vi "FRAS Module CdG.vi"(7 "error in":errorcluster, 8 "Imagette seuillée":i16[][](array[numeric]), 9 "inCdG[Pixels]":dbl[](array[numeric]), 10 "Mode CdG":T1(ring)=enum."Calcul CdG a") -> (0 "error out":errorcluster, 3 "CdGOut [Pixels]":dbl[](array[numeric]))   [LabVIEW 2020]
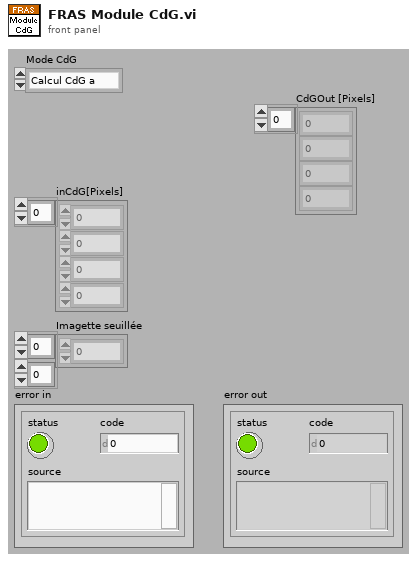
[diagram p1: front panel]
types:
  T1 = enum16{"Initialisation", "Calcul CdG a", "Calcul CdG b"}
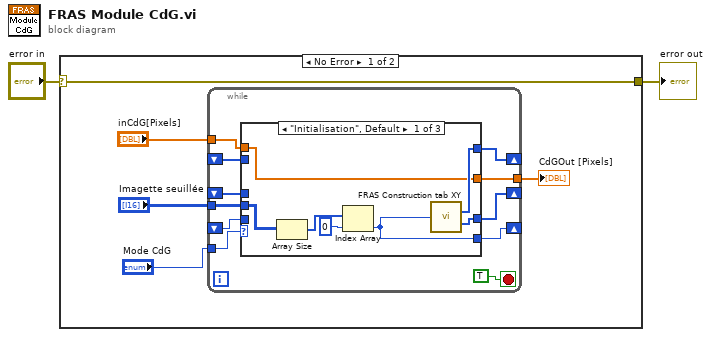
[diagram p0: block diagram]
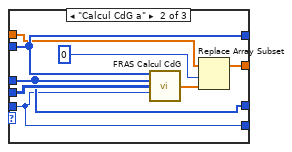
[diagram p2: hidden frame]
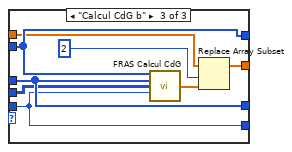
[diagram p3: hidden frame]
diagram:
  n1 = case shown="No Error" "error in" {
    selector: "error in" -> [w3 w42]
    tunnel: [w3 w42] -> w1
    frame No Error {
      n2 = while {
        tunnel: [w18] -> w7
        tunnel: "Imagette seuillée" -> [w17]
        tunnel: "Mode CdG" -> [w15]
        shift-right: [w14] -> _
        shift-left: _ -> [w12]
        shift-right: [w13] -> _
        shift-left: _ -> [w11]
        tunnel: "inCdG[Pixels]" -> [w10]
        shift-right: [w9] -> _
        shift-left: _ -> [w8]
        stop <- TRUE stop-if-true
        n3 = case shown="\"Initialisation\", Default" w15 {
          tunnel: [w19 w29 w37] -> w18
          tunnel: w17 -> [w21 w33 w35]
          tunnel: [w25 w32 w39] -> w14
          tunnel: [w24 w31 w38] -> w13
          tunnel: w12 -> [_ w32 w39]
          tunnel: w11 -> [_ w31 w38]
          tunnel: w10 -> [w19 w28 w36]
          tunnel: [w20 w26 w34] -> w9
          tunnel: w8 -> [_ w26 w34]
          frame "Initialisation", Default {
            n4 = Array Size(array=w21) -> (size(s)=w23:i32[])
            n5 = Index Array(array=w23, index=0) -> (element=w20:i32)
            n6 = call "FRAS Construction tab XY.vi"("Largeur cote"=w20) -> ("Tableau X"=w25:i32[], "Tableau Y"=w24:i32[])  [unwired: 13 out]
          }
          frame "Calcul CdG a" {
            n7 = call "FRAS Calcul CdG.vi"("Tableau X"=w32, "Tableau Y"=w31, "Imagette seuillée"=w33, "Largeur cote"=w26) -> ("CdG"=w30:sgl[])  [unwired: 11 out]
            n8 = Replace Array Subset(array=w28, new element=w30, index=0 ("indice")) -> (w29:dbl[])
          }
          frame "Calcul CdG b" {
            n9 = call "FRAS Calcul CdG.vi"("Tableau X"=w39, "Tableau Y"=w38, "Imagette seuillée"=w35, "Largeur cote"=w34) -> ("CdG"=w40:sgl[])  [unwired: 11 out]
            n10 = Replace Array Subset(array=w36, new element=w40, index=2 ("indice")) -> (w37:dbl[])
          }
        }
      }
      "CdGOut [Pixels]" <- w7
    }
    frame Error {
    }
  }
  "error out" <- w1
